vi "parseCallsData.vi"(11 "Array in":string[](array[string])) -> (3 "Array out":i32[](array[numeric]))   [LabVIEW 2017]
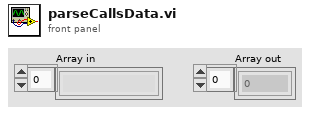
[diagram p1: front panel]
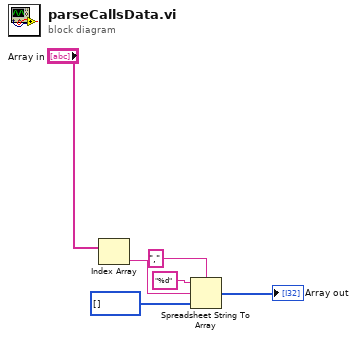
[diagram p0: block diagram]
diagram:
  n1 = Index Array(array="Array in") -> (element=w2:string)  [unwired: 1 in]
  n2 = Spreadsheet String To Array(delimiter (Tab)=",", format string="%d", spreadsheet string=w2, array type (2D Dbl)=i32[] []) -> (array=→"Array out":i32[])
